vi "ModbusWrite.vi"(0 "address":u16, 3 "holding register value":u16) -> (8 "error out":errorcluster)   [LabVIEW 2024]
uses:
  <vilib>/Modbus/master/Create Master Instance (TCP).vi
  <vilib>/Modbus/master/Modbus Master.lvclass
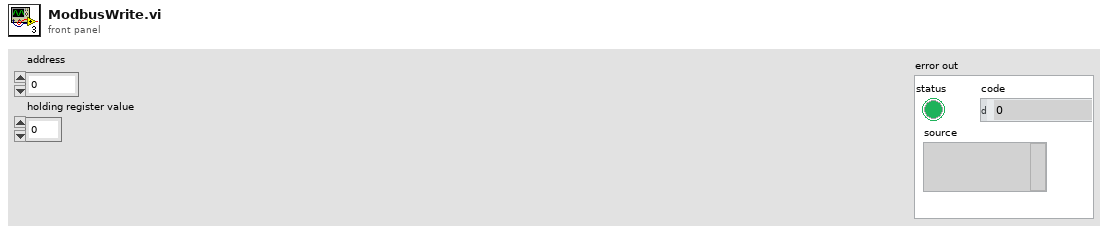
[diagram p1: front panel]
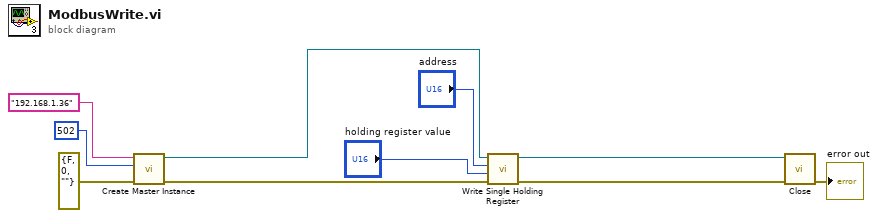
[diagram p0: block diagram]
diagram:
  n1 = call-poly <vilib>:"Create Master Instance.vi"("error in (no error)"=errorcluster {"status"=FALSE, "code"=0, "source"=""}, "port (502)"=u16 502, "address"="192.168.1.36") -> ("error out"=w7:errorcluster, "TCP master instance"=w6:refnum<class "Modbus Master.lvclass">)  [unwired: 7 in]
  n2 = call-dynamic "Write Single Holding Register.vi"("error in (no error)"=w7, "holding register value"="holding register value", "address"="address", "Modbus master in"=w6) -> ("error out"=w3:errorcluster, "Modbus master out"=w4:refnum<class "Modbus Master.lvclass">)  [unwired: 6 in]
  n3 = call-dynamic "Close.vi"("error in (no error)"=w3, "Modbus master in"=w4) -> ("error out"=→"error out":errorcluster)  [unwired: 9 in]
